vi "N6701A_STTOPowerOn.vi"(4 "Current Limit (amps)":dbl format="%^.3e", 5 "Inrush Current Factor (5x)":dbl=5.0, 6 "STTO Current Limit (amps)":dbl format="%^.3e", 7 "Voltage Level":dbl format="%^.3e", 8 "error in (no error)":errorcluster, 10 "Channel Name (1)":string="1", 11 "VISA resource name":refnum<visa-resource-name>) -> (0 "error out":errorcluster, 3 "VISA resource name out":refnum<visa-resource-name>)   [LabVIEW 2015]
doc: "This VI will set the Voltage taking into acount the polarity and the Current of the Power Supply\n\nThe input is an array of setting to allow the user to set all or one channel on as many devices as required"
uses:
  <instrlib>/Agilent N6700 Series/Agilent N6700 Series.lvlib
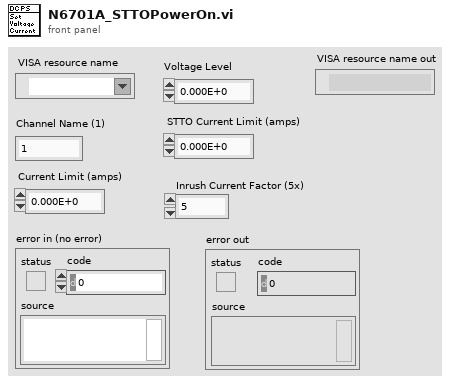
[diagram p1: front panel]
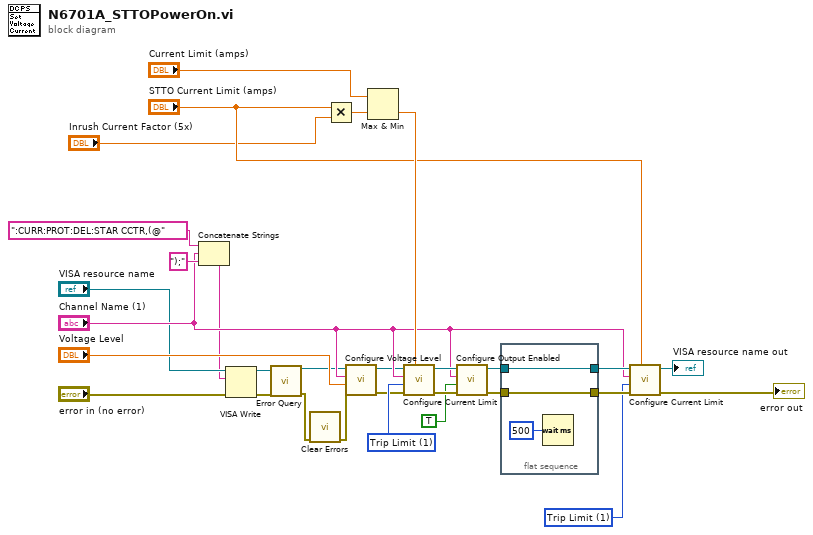
[diagram p0: block diagram]
diagram:
  w18 = 1 items=["Regulatory Limit", "Trip Limit"] ("Behavior (0: Regulatory Limit)")
  w26 = 1 items=["Regulatory Limit", "Trip Limit"] ("Behavior (0: Regulatory Limit)")
  n1 = Concatenate Strings(":CURR:PROT:DEL:STAR CCTR,(@" ("format string"), "Channel Name (1)", ");" ("string")) -> (w3:string)
  n2 = VISA Write(VISA resource name="VISA resource name", write buffer=w3, error in (no error)="error in (no error)") -> (VISA resource name out=w10:refnum<visa-resource-name>, error out=w9:errorcluster)  [unwired: 1 out]
  n3 = call <instrlib>:"Error Query.vi"("VISA resource name"=w10, "error in (no error)"=w9) -> ("VISA resource name out"=w6:refnum<visa-resource-name>, "error out"=w2:errorcluster)  [unwired: 10 in, 2 out]
  n4 = call <vilib>:"Clear Errors.vi"("error in (no error)"=w2) -> ("error out"=w1:errorcluster)  [unwired: 5 in, 1 out]
  n5 = Multiply(x="STTO Current Limit (amps)", y="Inrush Current Factor (5x)") -> (x*y=w28:dbl)
  n6 = call <instrlib>:"Configure Voltage Level.vi"("error in (no error)"=w1, "Level  (0.0 volts)"="Voltage Level", "Channel Name (1)"="Channel Name (1)", "VISA resource name"=w6) -> ("error out"=w7:errorcluster, "VISA resource name out"=w8:refnum<visa-resource-name>)  [unwired: 6 in]
  n7 = Max & Min(x="Current Limit (amps)", y=w28) -> (min(x,y)=w27:dbl)  [unwired: 1 out]
  n8 = call <instrlib>:"Configure Current Limit.vi"("Limit (0.0 amps)"=w27, "error in (no error)"=w7, "Behavior (0: Regulatory Limit)"=w26, "Channel Name (1)"="Channel Name (1)", "VISA resource name"=w8) -> ("error out"=w24:errorcluster, "VISA resource name out"=w25:refnum<visa-resource-name>)  [unwired: 5 in]
  n9 = call <instrlib>:"Configure Output Enabled.vi"("error in (no error)"=w24, "Enable Output (False)"=TRUE, "Channel Name (1)"="Channel Name (1)", "VISA resource name"=w25) -> ("error out"=w21:errorcluster, "VISA resource name out"=w22:refnum<visa-resource-name>)  [unwired: 6 in]
  n10 = flat-sequence {
    tunnel: w22 -> [w32]
    tunnel: w21 -> [w31]
    tunnel: [w32] -> w20
    tunnel: [w31] -> w19
    frame #0 {
      n11 = Wait (ms)(milliseconds to wait=u32 500) -> ()  [unwired: 1 out]
    }
  }
  n12 = call <instrlib>:"Configure Current Limit.vi"("Limit (0.0 amps)"="STTO Current Limit (amps)", "error in (no error)"=w19, "Behavior (0: Regulatory Limit)"=w18, "Channel Name (1)"="Channel Name (1)", "VISA resource name"=w20) -> ("error out"=→"error out":errorcluster, "VISA resource name out"=→"VISA resource name out":refnum<visa-resource-name>)  [unwired: 5 in]
